vi "RS_RF_init.vi"(1 "Initialize Instrument":u64, 2 "Inst_param":T1) -> ()   [LabVIEW 2013]
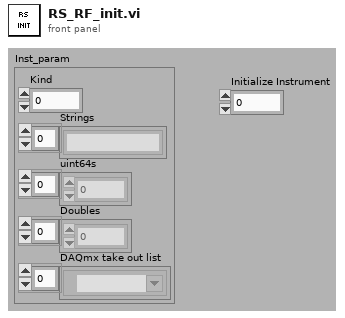
[diagram p1: front panel]
types:
  T1 = cluster{"Kind":u16, "Strings":string[], "uint64s":u64[], "Doubles":dbl[], "DAQmx take out list":refnum<k21>[]}
  T2 = enum16{"Frequency (GHz)", "Power (dBm)", "Pulse period (us)", "Pulse width (us)", "Pulse delay (us)", "Pulse modulation?", "Output on?", "Pulse source", "Pulse mode", "Trigger mode", "Ex trigger input slope", "External impedance"}[]
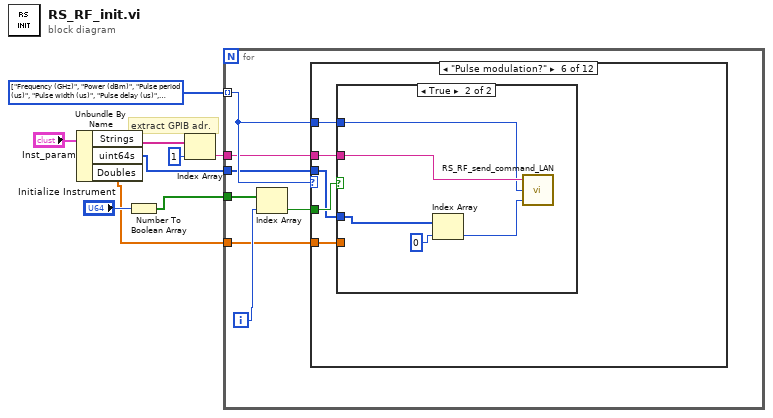
[diagram p0: block diagram]
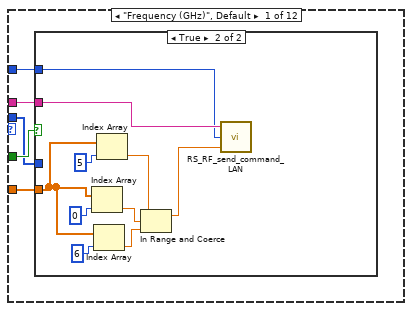
[diagram p2: hidden frame]
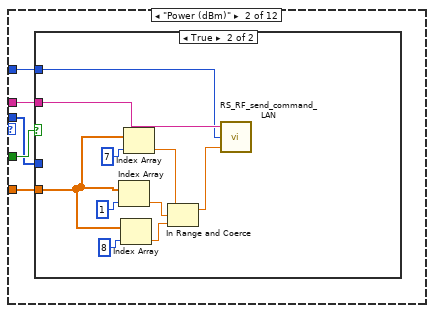
[diagram p4: hidden frame]
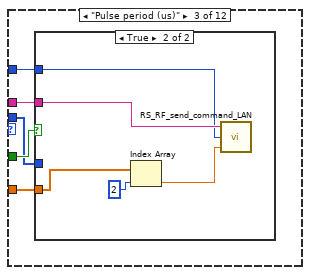
[diagram p6: hidden frame]
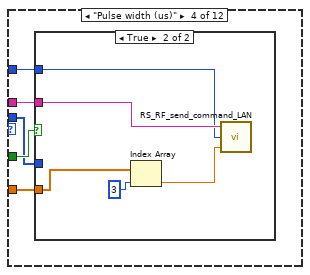
[diagram p8: hidden frame]
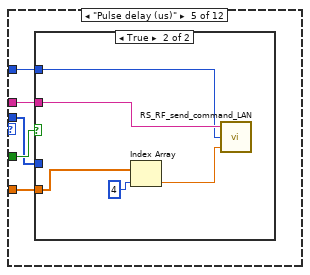
[diagram p10: hidden frame]
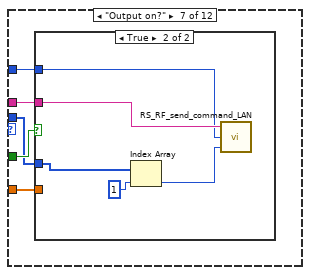
[diagram p13: hidden frame]
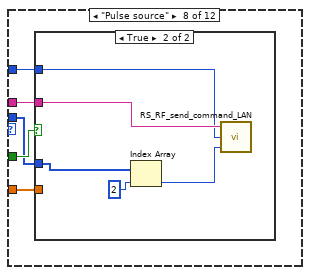
[diagram p15: hidden frame]
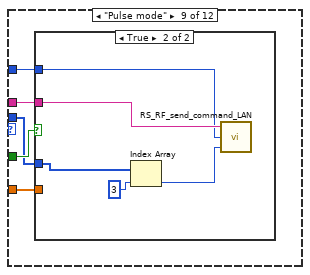
[diagram p17: hidden frame]
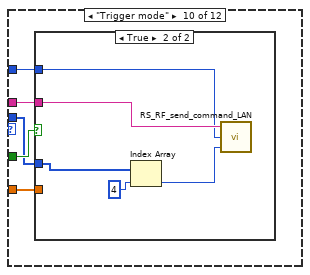
[diagram p19: hidden frame]
diagram:
  w9 = T2 [enum."Frequency (GHz)", enum."Power (dBm)", enum."Pulse period (us)", enum."Pulse width (us)", enum."Pulse delay (us)", enum."Pulse modulation?", enum."Output on?", enum."Pulse source", enum."Pulse mode", enum."Trigger mode", enum."Ex trigger input slope", enum."External impedance"] items=["Frequency (GHz)", "Power (dBm)", "Pulse period (us)", "Pulse width (us)", "Pulse delay (us)", "Pulse modulation?", "Output on?", "Pulse source", "Pulse mode", "Trigger mode", "Ex trigger input slope", "External impedance"]
  # "extract GPIB adr."
  n1 = Unbundle By Name("Inst_param") -> ("Strings"=w7:string[], "uint64s"=w2:u64[], "Doubles"=w1:dbl[])
  n2 = Number To Boolean Array(number="Initialize Instrument") -> (Boolean array=w3:bool[])
  n3 = Index Array(array=w7, index=1) -> (element=w5:string)
  n4 = for {
    tunnel: w9 -> [w14] mode=indexing
    tunnel: w5 -> [w12]
    tunnel: w3 -> [w16]
    tunnel: w2 -> [w11]
    tunnel: w1 -> [w10]
    i -> [w15]
    n5 = Index Array(array=w16, index=w15) -> (element=w13:bool)
    n6 = case shown="\"Pulse modulation?\"" w14 {
      tunnel: w14 -> [w19 w34 w49 w59 w69 w79 w89 w99 w109 w119 w129 w139]
      tunnel: w13 -> [w21 w36 w51 w61 w71 w81 w91 w101 w111 w121 w131 w141]
      tunnel: w12 -> [w20 w35 w50 w60 w70 w80 w90 w100 w110 w120 w130 w140]
      tunnel: w11 -> [w18 w33 w48 w58 w68 w78 w88 w98 w108 w118 w128 w138]
      tunnel: w10 -> [w17 w32 w47 w57 w67 w77 w87 w97 w107 w117 w127 w137]
      frame "Frequency (GHz)", Default {
        n7 = case shown="True" w21 {
          tunnel: w20 -> [_ w31]
          tunnel: w19 -> [_ w30]
          tunnel: w18 -> [_ _]
          tunnel: w17 -> [_ w26]
          frame False {
          }
          frame True {
            n8 = Index Array(array=w26, index=0) -> (element=w25:dbl)
            n9 = Index Array(array=w26, index=6) -> (element=w23:dbl)
            n10 = Index Array(array=w26, index=5) -> (element=w24:dbl)
            n11 = In Range and Coerce(upper limit=w24, x=w25, lower limit=w23) -> (coerced(x)=w22:dbl)  [unwired: 1 out]
            n12 = call "RS_RF_send_command_LAN.vi"("Value"=w22, "Parameter"=w30, "IP Address"=w31) -> ()  [unwired: 1 in]
          }
        }
      }
      frame "Power (dBm)" {
        n13 = case shown="True" w36 {
          tunnel: w35 -> [_ w46]
          tunnel: w34 -> [_ w45]
          tunnel: w33 -> [_ _]
          tunnel: w32 -> [_ w38]
          frame False {
          }
          frame True {
            n14 = Index Array(array=w38, index=1) -> (element=w41:dbl)
            n15 = Index Array(array=w38, index=8) -> (element=w39:dbl)
            n16 = Index Array(array=w38, index=7) -> (element=w40:dbl)
            n17 = In Range and Coerce(upper limit=w40, x=w41, lower limit=w39) -> (coerced(x)=w37:dbl)  [unwired: 1 out]
            n18 = call "RS_RF_send_command_LAN.vi"("Value"=w37, "Parameter"=w45, "IP Address"=w46) -> ()  [unwired: 1 in]
          }
        }
      }
      frame "Pulse period (us)" {
        n19 = case shown="True" w51 {
          tunnel: w50 -> [_ w56]
          tunnel: w49 -> [_ w55]
          tunnel: w48 -> [_ _]
          tunnel: w47 -> [_ w52]
          frame False {
          }
          frame True {
            n20 = Index Array(array=w52, index=2) -> (element=w53:dbl)
            n21 = call "RS_RF_send_command_LAN.vi"("Value"=w53, "Parameter"=w55, "IP Address"=w56) -> ()  [unwired: 1 in]
          }
        }
      }
      frame "Pulse width (us)" {
        n22 = case shown="True" w61 {
          tunnel: w60 -> [_ w66]
          tunnel: w59 -> [_ w65]
          tunnel: w58 -> [_ _]
          tunnel: w57 -> [_ w62]
          frame False {
          }
          frame True {
            n23 = Index Array(array=w62, index=3) -> (element=w63:dbl)
            n24 = call "RS_RF_send_command_LAN.vi"("Value"=w63, "Parameter"=w65, "IP Address"=w66) -> ()  [unwired: 1 in]
          }
        }
      }
      frame "Pulse delay (us)" {
        n25 = case shown="True" w71 {
          tunnel: w70 -> [_ w76]
          tunnel: w69 -> [_ w75]
          tunnel: w68 -> [_ _]
          tunnel: w67 -> [_ w72]
          frame False {
          }
          frame True {
            n26 = Index Array(array=w72, index=4) -> (element=w73:dbl)
            n27 = call "RS_RF_send_command_LAN.vi"("Value"=w73, "Parameter"=w75, "IP Address"=w76) -> ()  [unwired: 1 in]
          }
        }
      }
      frame "Pulse modulation?" {
        n28 = case shown="True" w81 {
          tunnel: w80 -> [_ w86]
          tunnel: w79 -> [_ w85]
          tunnel: w78 -> [_ w82]
          tunnel: w77 -> [_ _]
          frame False {
          }
          frame True {
            n29 = Index Array(array=w82, index=0) -> (element=w83:u64)
            n30 = call "RS_RF_send_command_LAN.vi"("Value"=w83, "Parameter"=w85, "IP Address"=w86) -> ()  [unwired: 1 in]
          }
        }
      }
      frame "Output on?" {
        n31 = case shown="True" w91 {
          tunnel: w90 -> [_ w96]
          tunnel: w89 -> [_ w95]
          tunnel: w88 -> [_ w92]
          tunnel: w87 -> [_ _]
          frame False {
          }
          frame True {
            n32 = Index Array(array=w92, index=1) -> (element=w93:u64)
            n33 = call "RS_RF_send_command_LAN.vi"("Value"=w93, "Parameter"=w95, "IP Address"=w96) -> ()  [unwired: 1 in]
          }
        }
      }
      frame "Pulse source" {
        n34 = case shown="True" w101 {
          tunnel: w100 -> [_ w106]
          tunnel: w99 -> [_ w105]
          tunnel: w98 -> [_ w102]
          tunnel: w97 -> [_ _]
          frame False {
          }
          frame True {
            n35 = Index Array(array=w102, index=2) -> (element=w103:u64)
            n36 = call "RS_RF_send_command_LAN.vi"("Value"=w103, "Parameter"=w105, "IP Address"=w106) -> ()  [unwired: 1 in]
          }
        }
      }
      frame "Pulse mode" {
        n37 = case shown="True" w111 {
          tunnel: w110 -> [_ w116]
          tunnel: w109 -> [_ w115]
          tunnel: w108 -> [_ w112]
          tunnel: w107 -> [_ _]
          frame False {
          }
          frame True {
            n38 = Index Array(array=w112, index=3) -> (element=w113:u64)
            n39 = call "RS_RF_send_command_LAN.vi"("Value"=w113, "Parameter"=w115, "IP Address"=w116) -> ()  [unwired: 1 in]
          }
        }
      }
      frame "Trigger mode" {
        n40 = case shown="True" w121 {
          tunnel: w120 -> [_ w126]
          tunnel: w119 -> [_ w125]
          tunnel: w118 -> [_ w122]
          tunnel: w117 -> [_ _]
          frame False {
          }
          frame True {
            n41 = Index Array(array=w122, index=4) -> (element=w123:u64)
            n42 = call "RS_RF_send_command_LAN.vi"("Value"=w123, "Parameter"=w125, "IP Address"=w126) -> ()  [unwired: 1 in]
          }
        }
      }
      frame "Ex trigger input slope" {
        n43 = case shown="True" w131 {
          tunnel: w130 -> [_ w136]
          tunnel: w129 -> [_ w135]
          tunnel: w128 -> [_ w132]
          tunnel: w127 -> [_ _]
          frame False {
          }
          frame True {
            n44 = Index Array(array=w132, index=5) -> (element=w133:u64)
            n45 = call "RS_RF_send_command_LAN.vi"("Value"=w133, "Parameter"=w135, "IP Address"=w136) -> ()  [unwired: 1 in]
          }
        }
      }
      frame "External impedance" {
        n46 = case shown="True" w141 {
          tunnel: w140 -> [_ w146]
          tunnel: w139 -> [_ w145]
          tunnel: w138 -> [_ w142]
          tunnel: w137 -> [_ _]
          frame False {
          }
          frame True {
            n47 = Index Array(array=w142, index=6) -> (element=w143:u64)
            n48 = call "RS_RF_send_command_LAN.vi"("Value"=w143, "Parameter"=w145, "IP Address"=w146) -> ()  [unwired: 1 in]
          }
        }
      }
    }
  }
